vi "solar_voy_def Rename Channels.vi"(6 "Replace Existing? (T)":bool=TRUE, 7 "Parameter/Item Name":string, 8 "error in (no error)":errorcluster, 9 "Values":string[](array[string]), 10 "States":string[](array[string]), 11 "Packets in":T1[](array[typedef]) {"last_time" format="%<%H:%M:%S%3u %m/%d/%y>T"}) -> (0 "error out":errorcluster, 3 "Packets out":T1[](array[typedef]) {"last_time" format="%<%H:%M:%S%3u %m/%d/%y>T"})   [LabVIEW 2018]
doc: "This adds states to the parameter/item name if found. By default, this replaces any existing states registered with the packet. This is useful for specifying channel names at run-time."
uses:
  solar_voy_def_ctl MODIFIERS CONVERSION.ctl
  solar_voy_def_ctl MODIFIERS STATE.ctl
  solar_voy_def_ctl MODIFIERS UNITS.ctl
  solar_voy_def_ctl MODIFIERS LIMITS.ctl
  solar_voy_def_ctl MODIFIERS.ctl
  solar_voy_def_ctl ITEM TYPE.ctl
  type/solar_type Item Type.ctl
  solar_voy_def_ctl ITEM.ctl
  solar_voy_def_ctl PACKET_ID.ctl
  solar_voy_def_ctl PACKET.ctl
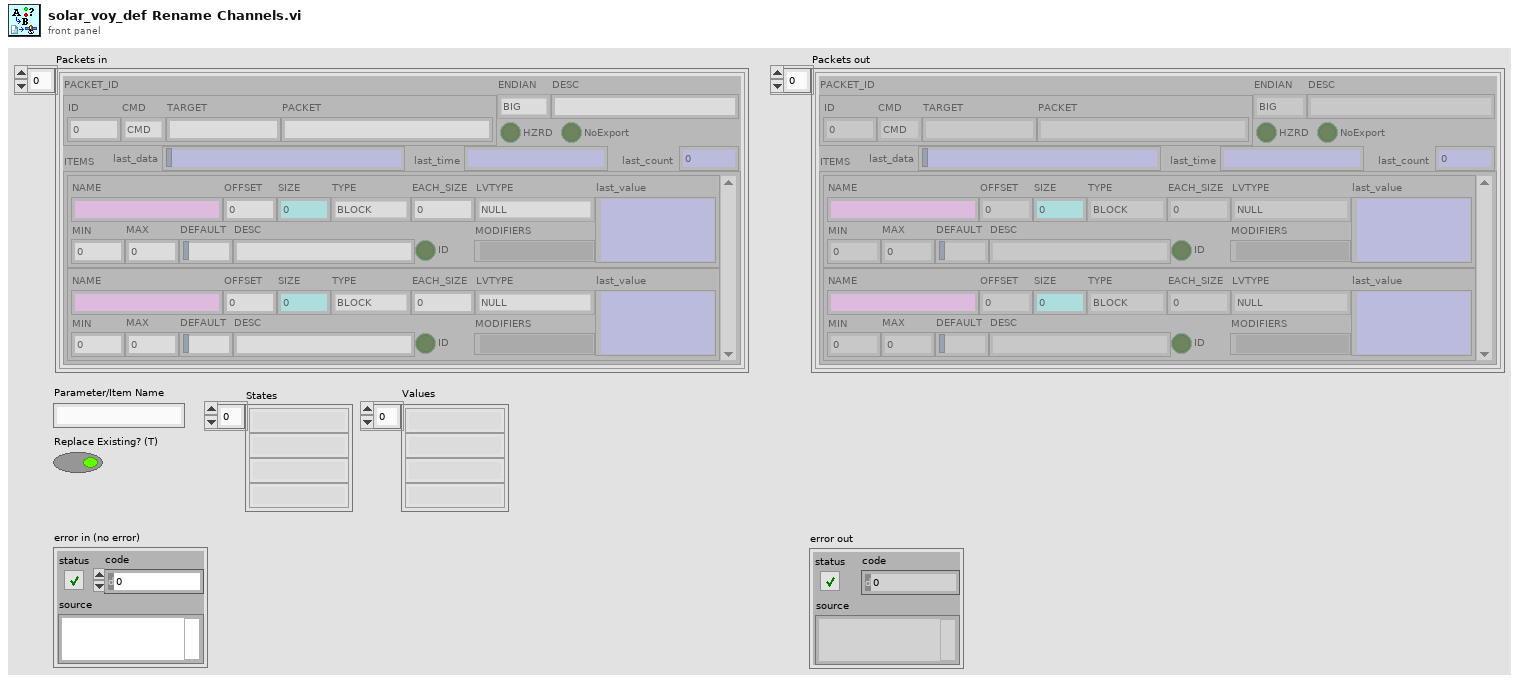
[diagram p1: front panel]
types:
  T1 = typedef "solar_voy_def_ctl PACKET.ctl" = cluster{"PACKET_ID":T2, "ENDIAN":enum8{"BIG", "LITTLE"}, "DESC":string, "HZRD":bool, "ITEMS":T3[], "NoExport":bool, "last_time":timestamp, "last_count":u32, "last_data":string}
  T2 = typedef "solar_voy_def_ctl PACKET_ID.ctl" = cluster{"ID":u16, "CMD":enum8{"CMD", "TLM"}, "TARGET":string, "PACKET":string}
  T3 = typedef "solar_voy_def_ctl ITEM.ctl" = cluster{"NAME":string, "OFFSET":i32, "SIZE":i32, "TYPE":T4, "EACH_SIZE":i32, "LVTYPE":T5, "MIN":dbl, "MAX":dbl, "DEFAULT":string, "DESC":string, "ID":bool, "MODIFIERS":variant, "last_value":variant}
  T4 = typedef "solar_voy_def_ctl ITEM TYPE.ctl" = enum8{"BLOCK", "INT", "UINT", "FLOAT", "STRING"}
  T5 = typedef "solar_type Item Type.ctl" = enum16{"NULL", "UNKNOWN", "CLUSTER", "I8", "I16", "I32", "I64", "U8", "U16", "U32", "U64", "U8_ENUM", "U16_ENUM", "U32_ENUM", "SGL", "DBL", "BOOLEAN", "STRING", "PATH", "VISA", "TAG", "TIME", "I8_1D", "I16_1D", "I32_1D", "I64_1D", "U8_1D", "U16_1D", "U32_1D", "U64_1D", "U8_ENUM_1D", "U16_ENUM_1D", "U32_ENUM_1D", "SGL_1D", "DBL_1D", "BOOLEAN_1D", "STRING_1D", "PATH_1D", "VISA_1D", "TAG_1D", "TIME_1D", "I8_2D", "I16_2D", "I32_2D", "I64_2D", "U8_2D", "U16_2D", "U32_2D", "U64_2D", "U8_ENUM_2D", "U16_ENUM_2D", "U32_ENUM_2D", "SGL_2D", "DBL_2D", "BOOLEAN_2D", "STRING_2D", "PATH_2D", "VISA_2D", "TAG_2D", "TIME_2D"}
  T6 = typedef "solar_voy_def_ctl MODIFIERS STATE.ctl" = cluster{"KEY":string, "VALUE":string, "COLOR":string, "DESC":string, "HZRD":bool}
  T7 = typedef "solar_voy_def_ctl MODIFIERS.ctl" = cluster{"LIMITS":T8, "UNITS":T9, "STATES":T6[], "CONVERSION":T10, "FORMAT":string, "REQUIRED":bool, "META":string[][]}
  T8 = typedef "solar_voy_def_ctl MODIFIERS LIMITS.ctl" = cluster{"NAME":string, "PERSIST":i32, "EN":bool, "RED_LO":dbl, "YEL_LO":dbl, "YEL_HI":dbl, "RED_HI":dbl, "GRN_LO":dbl, "GRN_HI":dbl, "FILENAME":string, "ARGS":string}
  T9 = typedef "solar_voy_def_ctl MODIFIERS UNITS.ctl" = cluster{"FULL":string, "ABV":string}
  T10 = typedef "solar_voy_def_ctl MODIFIERS CONVERSION.ctl" = cluster{"GENERIC":string, "FILENAME":string, "ARGS":string, "POLYS":cluster{"SEG":bool, "POLY":dbl[]}[]}
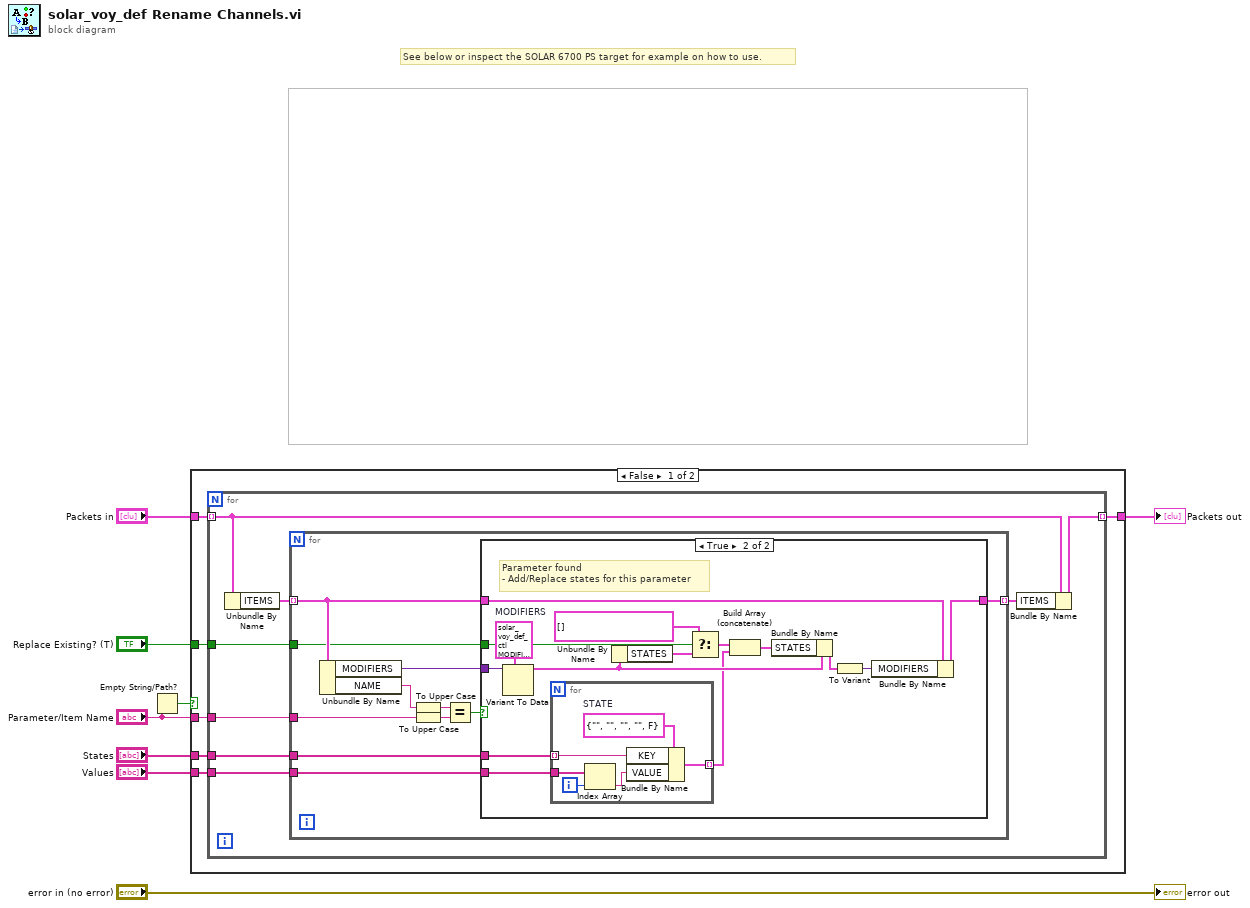
[diagram p0: block diagram]
diagram:
  # "See below or inspect the SOLAR 6700 PS target for example on how to use."
  n1 = Empty String/Path?(string/path="Parameter/Item Name") -> (empty?=w2:bool)
  n2 = case shown="False" w2 {
    tunnel: "Packets in" -> [w14 w56]
    tunnel: [w13 w56] -> w7
    tunnel: "Parameter/Item Name" -> [w12 _]
    tunnel: "States" -> [w11 _]
    tunnel: "Replace Existing? (T)" -> [w10 _]
    tunnel: "Values" -> [w9 _]
    frame False {
      n3 = for {
        tunnel: w14 -> [w22] mode=indexing
        tunnel: [w20] -> w13 mode=indexing
        tunnel: w12 -> [w18]
        tunnel: w11 -> [w17]
        tunnel: w10 -> [w16]
        tunnel: w9 -> [w15]
        n4 = Unbundle By Name(w22) -> ("ITEMS"=w21:T3[])
        n5 = for {
          tunnel: w21 -> [w33] mode=indexing
          tunnel: [w27] -> w19 mode=indexing
          tunnel: w18 -> [w28]
          tunnel: w17 -> [w25]
          tunnel: w16 -> [w24]
          tunnel: w15 -> [w23]
          n6 = Unbundle By Name(w33) -> ("MODIFIERS"=w32:variant, "NAME"=w31:string)
          n7 = To Upper Case(1:w31) -> (0:w30:string)
          n8 = To Upper Case(1:w28) -> (0:w29:string)
          n9 = Equal?(x=w30, y=w29) -> (x = y?=w26:bool)
          n10 = case shown="True" w26 {
            tunnel: w33 -> [w34 w49]
            tunnel: w32 -> [_ w48]
            tunnel: [w34 w44] -> w27
            tunnel: w25 -> [_ w37]
            tunnel: w24 -> [_ w36]
            tunnel: w23 -> [_ w35]
            frame False {
            }
            frame True {
              w47 = T7 {"LIMITS"={"NAME"="", "PERSIST"=0, "EN"=FALSE, "RED_LO"=0.0, "YEL_LO"=0.0, "YEL_HI"=0.0, "RED_HI"=0.0, "GRN_LO"=0.0, "GRN_HI"=0.0, "FILENAME"="", "ARGS"=""}, "UNITS"={"FULL"="", "ABV"=""}, "STATES"=[], "CONVERSION"={"GENERIC"="", "FILENAME"="", "ARGS"="", "POLYS"=[]}, "FORMAT"="", "REQUIRED"=FALSE, "META"=[]}  # MODIFIERS
              # "Parameter found\n- Add/Replace states for this parameter"
              n11 = Variant To Data(type=w47, Variant=w48) -> (data=w46:T7)  [unwired: 1 in, 1 out]
              n12 = for {
                tunnel: [w54] -> w38 mode=indexing
                tunnel: w37 -> [w53] mode=indexing
                tunnel: w35 -> [w52]
                i -> [w50]
                w55 = T6 {"KEY"="", "VALUE"="", "COLOR"="", "DESC"="", "HZRD"=FALSE}  # STATE
                n13 = Index Array(array=w52, index=w50) -> (element=w51:string)
                n14 = Bundle By Name(cluster=w55, "KEY"=w53, "VALUE"=w51) -> (w54:T6)
              }
              n15 = Unbundle By Name(w46) -> ("STATES"=w41:T6[])
              n16 = Select(t=T6[] [], s=w36, f=w41) -> (s? t:f=w40:T6[])
              n17 = Build Array (concatenate)(w40, w38) -> (w45:T6[])
              n18 = Bundle By Name(cluster=w46, "STATES"=w45) -> (w43:T7)
              n19 = To Variant(anything=w43) -> (Variant=w42:variant)
              n20 = Bundle By Name(cluster=w49, "MODIFIERS"=w42) -> (w44:T3)
            }
          }
        }
        n21 = Bundle By Name(cluster=w22, "ITEMS"=w19) -> (w20:T1)
      }
    }
    frame True {
    }
  }
  "Packets out" <- w7
  "error out" <- "error in (no error)"
